vi "Read basePoint.vi"(8 "error in (no error)":errorcluster, 11 "AlignSkill in":refnum<class "AlignSkill.lvclass">) -> (0 "error out":errorcluster, 2 "basePoint":dbl[](array[numeric]), 3 "AlignSkill out":refnum<class "AlignSkill.lvclass">)   [LabVIEW 2023, in "AlignSkill.lvclass"]
uses:
  AlignSkill.lvclass
  AlignSkill.lvclass/AlignSkill.ctl
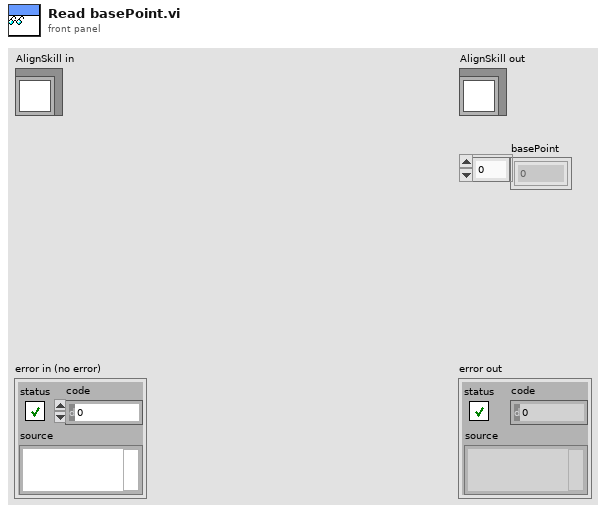
[diagram p1: front panel]
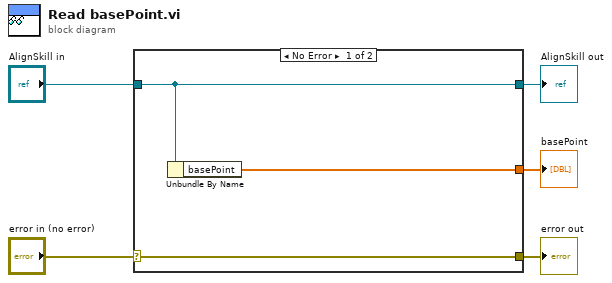
[diagram p0: block diagram]
diagram:
  n1 = case shown="No Error" "error in (no error)" {
    selector: "error in (no error)" -> [w8 w9]
    tunnel: [w8 w9] -> w4
    tunnel: [w7 w10] -> w2
    tunnel: "AlignSkill in" -> [w7 w10]
    tunnel: [w6 _] -> w1
    frame No Error {
      n2 = Unbundle By Name(w7) -> ("basePoint"=w6:dbl[])
    }
    frame Error {
    }
  }
  "error out" <- w4
  "AlignSkill out" <- w2
  "basePoint" <- w1
